vi "INIScoreFile Check Score.vi"(8 "error in (no error)":errorcluster, 10 "Score":u32, 11 "INIScoreFile in":refnum<class "INIScoreFile.lvclass">) -> (0 "error out":errorcluster, 2 "Is High?":bool, 3 "INIScoreFile out":refnum<class "INIScoreFile.lvclass">)   [LabVIEW 2020, in "INIScoreFile.lvclass"]
uses:
  INIScoreFile.lvclass
  INIScoreFile.lvclass/INIScoreFile.ctl
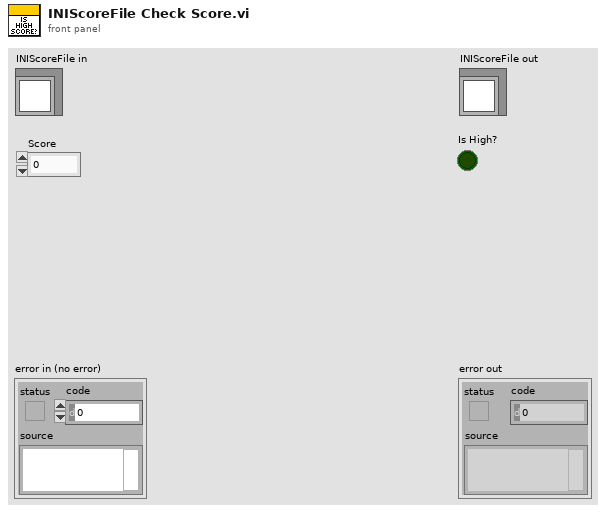
[diagram p1: front panel]
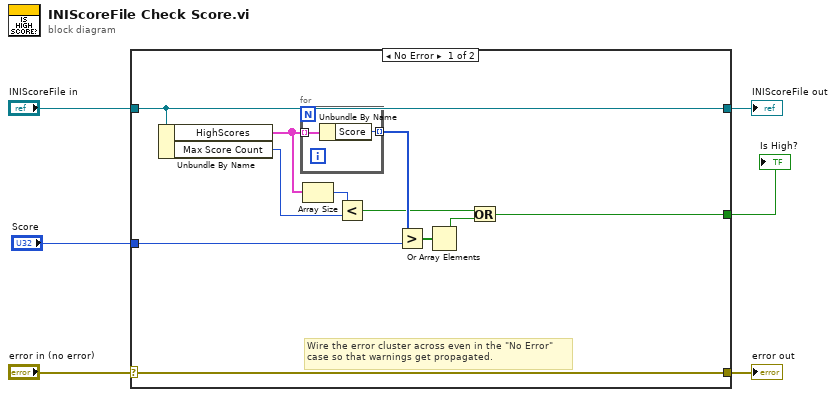
[diagram p0: block diagram]
diagram:
  n1 = case shown="No Error" "error in (no error)" {
    selector: "error in (no error)" -> [w17 w21]
    tunnel: [w17 w21] -> w5
    tunnel: [w16 w20] -> w3
    tunnel: "INIScoreFile in" -> [w16 w20]
    tunnel: "Score" -> [w11 _]
    tunnel: [w7 _] -> w1
    frame No Error {
      # "Wire the error cluster across even in the \"No Error\"\ncase so that warnings get propagated."
      n2 = Unbundle By Name(w16) -> ("HighScores"=w15:cluster{"Score":u32, "Name":string}[], "Max Score Count"=w13:i32)
      n3 = for {
        tunnel: w15 -> [w19] mode=indexing
        tunnel: [w18] -> w12 mode=indexing
        n4 = Unbundle By Name(w19) -> ("Score"=w18:u32)
      }
      n5 = Array Size(array=w15) -> (size(s)=w14:i32)
      n6 = Less?(x=w14, y=w13) -> (x < y?=w8:bool)
      n7 = Greater?(x=w12, y=w11) -> (0:w10:bool[])
      n8 = Or Array Elements(Boolean array=w10) -> (logical OR=w9:bool)
      n9 = Or(x=w8, y=w9) -> (x .or. y?=w7:bool)
    }
    frame Error {
    }
  }
  "error out" <- w5
  "INIScoreFile out" <- w3
  "Is High?" <- w1
